vi "Repair.vi"() -> ()   [LabVIEW 2019]
uses:
  Control 3.ctl
  Control 1.ctl
  <vilib>/Analysis/3filter.llb/Filter Passband Type.ctl
  <vilib>/Analysis/5stat.llb/RMS (DBL).vi
  <vilib>/Waveform/WDTOps.llb/WDT Append Waveforms DBL.vi
  <vilib>/Analysis/3filter.llb/Butterworth Filter (DBL).vi
  <vilib>/Analysis/NI_AALPro.lvlib
  <vilib>/Analysis/NI_AALBase.lvlib
panel:
  out "1/x":dbl
  out "Numeric":dbl
  out "XY Graph":cluster{dbl[], "Vstupní pole":dbl[]}(graph)
  out "Prubehy RMS":cluster{"rms value":dbl}(graph)
  out "Perioda ze spektra.":dbl
  out "Urms":dbl format="%0.2f"
  out "Perioda z pruchodu nulou.":dbl
  out "Frekvence z pruchodu nulou.":dbl
  out "Frekvence ze spektra.":i32
  out "Spektrum prevzorkovaneho signalu":cluster{dbl[], dbl[]}(graph)
  out "Prevzorkovany signal":waveform(dbl)(graph)
  in  "Napetovy treshold":dbl=10.0
  in  "Sirka okna (ms)":i32(listbox)=1
  in  "Offset":dbl format="%0.2p"
  in  "Amplituda sumu":T1
  in  "Amplituda":dbl=1.0 format="%0.2p"
  in  "Frekvence":dbl=10.0 format="%0.2p"
  out "Signal z generatoru":waveform(dbl)(graph)
  in  "stop":bool
  # "Parametry generatoru signalu"
  # "Hide!"
  # "Parametry navzorkovaneho signalu"
  # "Parametry prevzorkovaneho signalu"
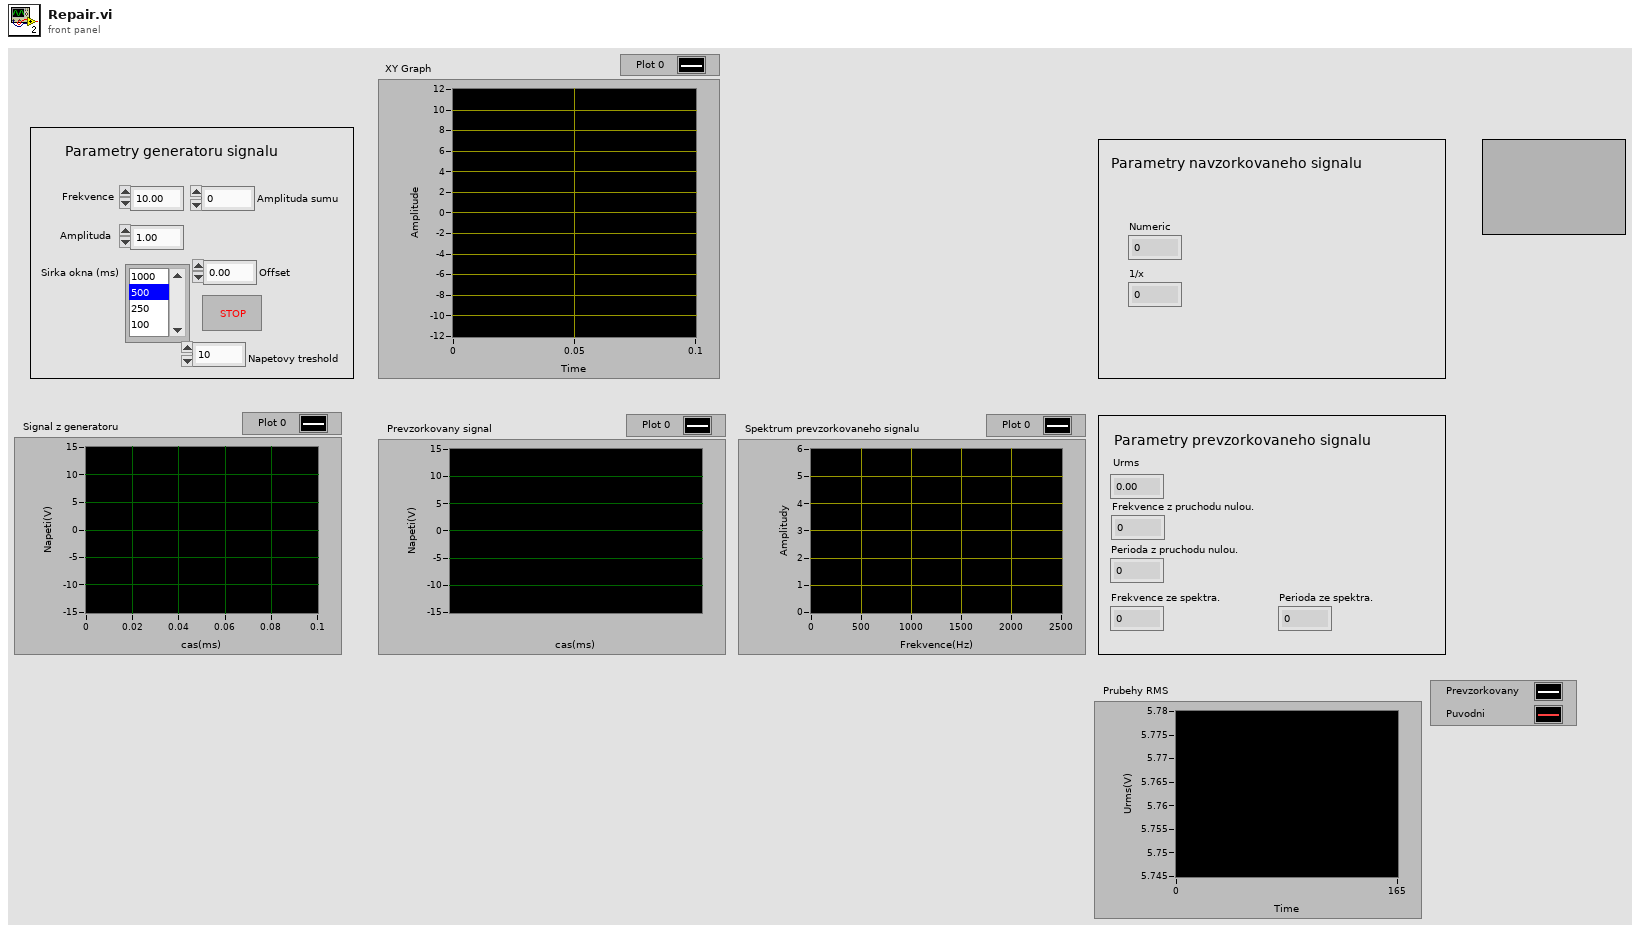
[diagram p1: front panel]
types:
  T1 = typedef "Control 3.ctl" = dbl
  T2 = enum16{"open", "open or create", "create or replace", "create", "open (read-only)"}
  T3 = cluster{"Waveform":waveform(dbl), "Waveform":waveform(dbl), "Waveform":waveform(dbl), "seconds since 1Jan1904":timestamp, bool, bool}
  T4 = typedef "Control 1.ctl" = dbl
  T5 = cluster{"name (unnamed)":string, "Variant":variant}
  T6 = typedef "NI_AALBase.lvlib/Filter Passband Type.ctl" = enum32{"Lowpass", "Highpass", "Bandpass", "Bandstop"}
  T7 = cluster{waveform(dbl), waveform(dbl), waveform(dbl), "seconds since 1Jan1904":timestamp, bool, bool}
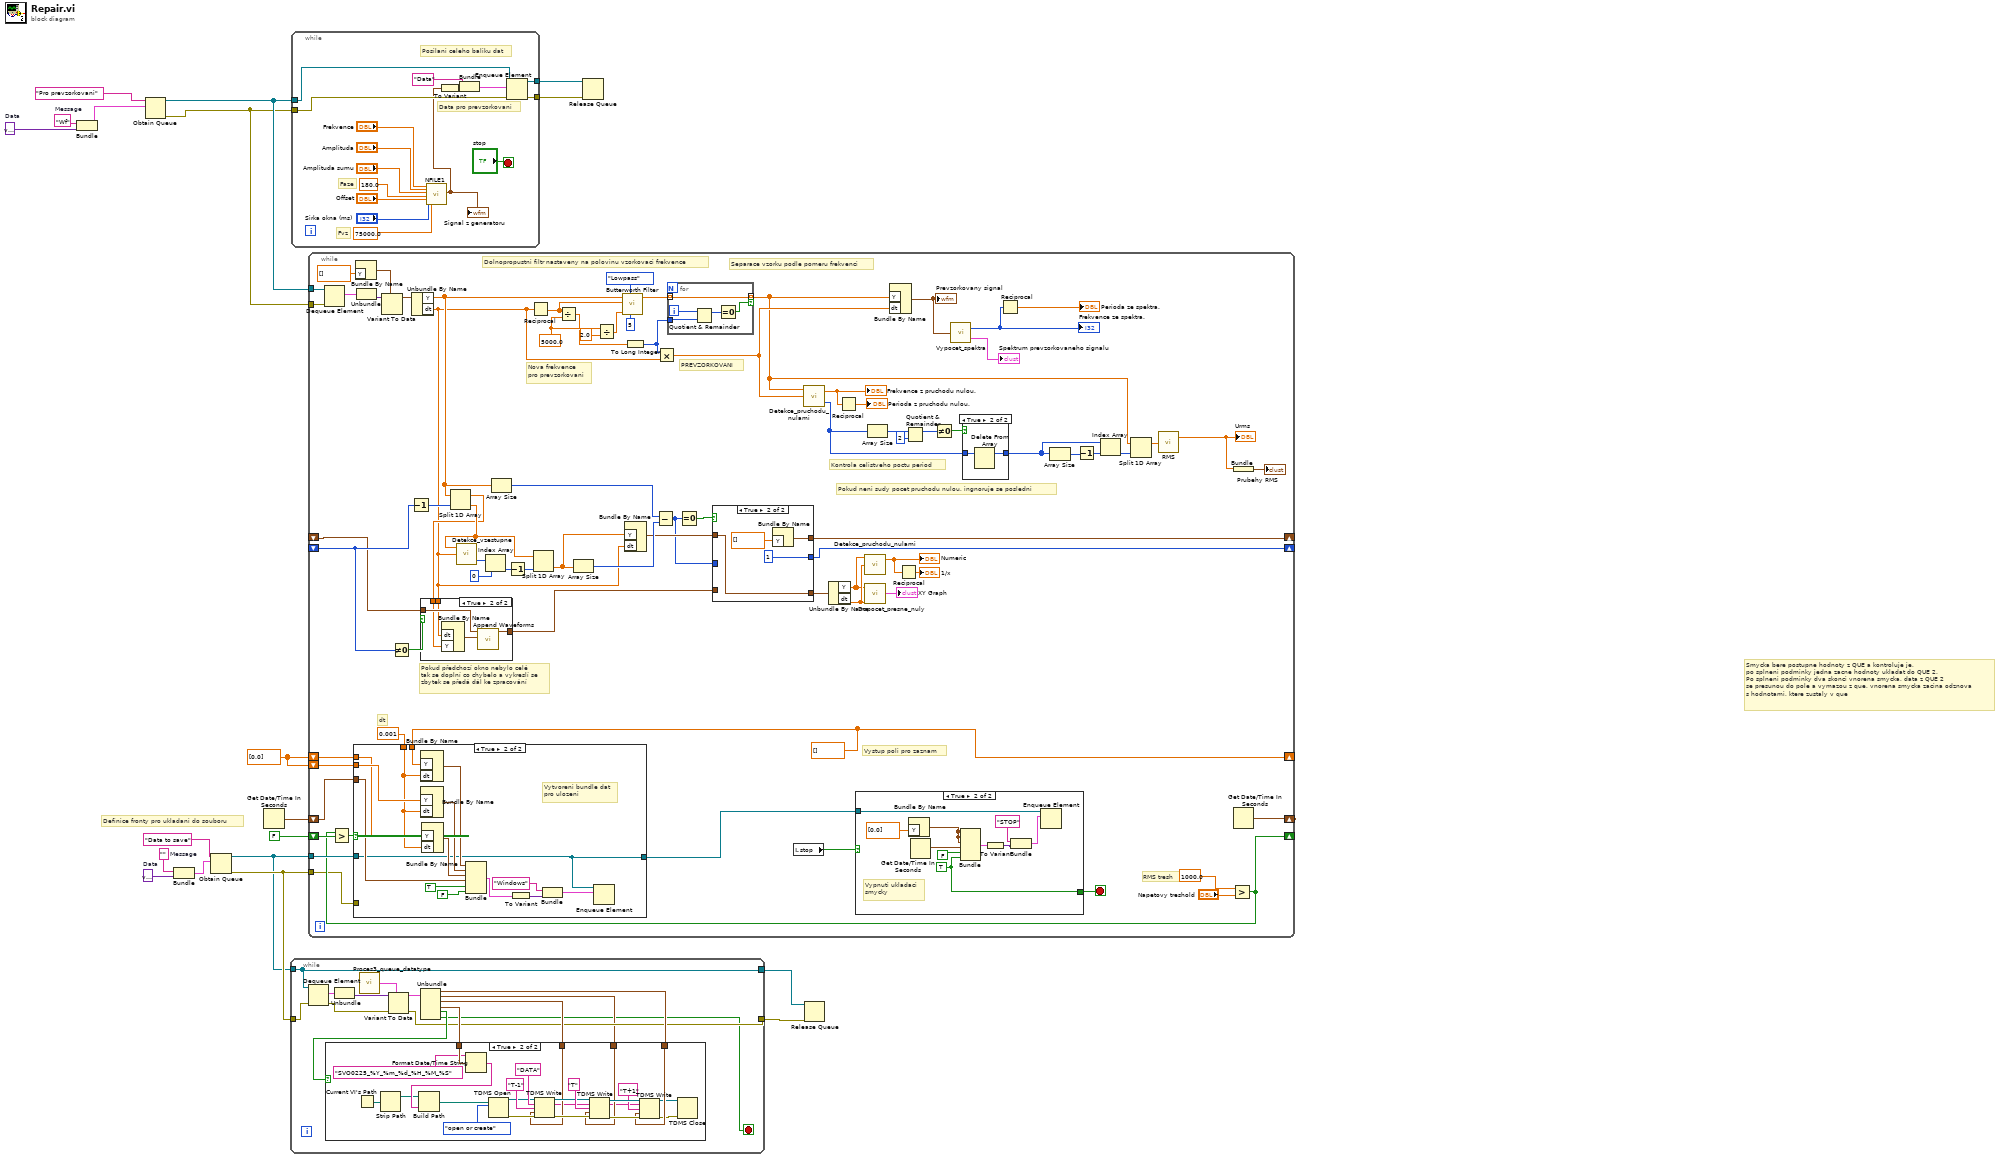
[diagram p0: block diagram]
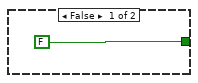
[diagram p5: hidden frame]
diagram:
  w4 = dbl[] [0.0]
  w3 = variant  # Data
  w8 = "Wf"  # Message
  w17 = variant  # Data
  w18 = ""  # Message
  # "Definice fronty pro ukladani do souboru"
  # "Smycka bere postupne hodnoty z QUE a kontroluje je,\npo splneni podminky jedna zacne hodnoty ukladat do QUE 2.\nPo splneni podminky dva skonci vnorena smycka, data z QUE 2 \nse presunou do pole a vymazou z que, vnorena smycka zacina odznova\ns hodnotami, ktere zustaly v que"
  n1 = Bundle("Message"=w8, "Data"=w3) -> (w7:cluster{"Message":string, "Data":variant})  [unwired: 1 in]
  n2 = Obtain Queue(name (unnamed)="Pro prevzorkovani", element data type=w7) -> (queue out=w10:refnum<queue>, error out=w9:errorcluster)  [unwired: 3 in, 1 out]
  n3 = Bundle("Message"=w18, "Data"=w17) -> (w16:cluster{"Message":string, "Data":variant})  [unwired: 1 in]
  n4 = Obtain Queue(name (unnamed)="Data to save", element data type=w16) -> (queue out=w13:refnum<queue>, error out=w14:errorcluster)  [unwired: 3 in, 1 out]
  n5 = Get Date/Time In Seconds() -> (seconds since 1Jan1904=w5:timestamp)
  n6 = while {
    tunnel: w14 -> [w24]
    tunnel: w13 -> [w29]
    tunnel: [w29] -> w12
    tunnel: [w22] -> w11
    stop <- w20 stop-if-true
    n7 = Dequeue Element(queue=w29, error in (no error)=w24) -> (element=w33:cluster{"Message":string, "Data":variant}, error out=w23:errorcluster)  [unwired: 1 in, 2 out]
    n8 = Unbundle(w33) -> ("Data"=w32:variant)  [unwired: 1 out]
    n9 = call "Proces3_queue_datatype.vi"() -> ("output cluster"=w31:T3)  [unwired: 1 in]
    n10 = Variant To Data(error in=w23, type=w31, Variant=w32) -> (data=w30:T3, error out=w22:errorcluster)
    n11 = Unbundle(w30) -> ("Waveform"=w28:waveform(dbl), "Waveform"=w21:waveform(dbl), "Waveform"=w25:waveform(dbl), "seconds since 1Jan1904"=w27:timestamp, w26:bool, w20:bool)
    n12 = case shown="True" w26 {
      tunnel: w28 -> [_ w46]
      tunnel: w27 -> [_ w45]
      tunnel: w25 -> [_ w39]
      tunnel: w21 -> [_ w38]
      frame False {
      }
      frame True {
        n13 = Current VI's Path() -> (path=w57:path)
        n14 = Strip Path(path=w57) -> (stripped path=w34:path)  [unwired: 1 out]
        n15 = Format Date/Time String(time format string (%c)="SVO0225_%Y_%m_%d_%H_%M_%S", seconds (now)=w45) -> (date/time string=w56:string)  [unwired: 1 in]
        n16 = Build Path(base path=w34, name or relative path=w56) -> (appended path=w55:path)
        n17 = TDMS Open(10:T2."open or create" ("operation (0:open)"), 11:w55) -> (0:w50:errorcluster, 3:w51:refnum<k34>)  [unwired: 5 in]
        n18 = TDMS Write(0:w51, 5:"DATA" ("group name in (Untitled)"), 7:"T-1", 9:w39, 11:w50) -> (4:w40:refnum<k34>, 6:w37:string, 15:w49:errorcluster)  [unwired: 1 in, 1 out]
        n19 = TDMS Write(0:w40, 5:w37, 7:"T", 9:w38, 11:w49) -> (4:w41:refnum<k34>, 6:w35:string, 15:w47:errorcluster)  [unwired: 1 in, 1 out]
        n20 = TDMS Write(0:w41, 5:w35, 7:"T+1", 9:w46, 11:w47) -> (4:w43:refnum<k34>, 15:w44:errorcluster)  [unwired: 1 in, 2 out]
        n21 = TDMS Close(8:w44, 11:w43) -> ()  [unwired: 2 out]
      }
    }
  }
  n22 = while {
    tunnel: w10 -> [w65]
    tunnel: w9 -> [w64]
    tunnel: [w59] -> w2
    tunnel: [w58] -> w1
    stop <- "stop" stop-if-true
    # "Posilani celeho baliku dat"
    # "Data pro prevzorkovani"
    # "Fvz"
    # "Faze"
    n23 = call "NFILE1.vi"("Frekvence"="Frekvence", "Amplituda"="Amplituda", "Amplituda sumu"="Amplituda sumu", "Fáze"=180.0, "Offset"="Offset", "Sirka okna (ms)"="Sirka okna (ms)", "Fvz"=T4 75000.0) -> ("Waveform Graph"=w61:waveform(dbl))  [unwired: 12 in]
    "Signal z generatoru" <- w61
    n24 = To Variant(anything=w61) -> (Variant=w62:variant)
    n25 = Bundle("name (unnamed)"="Data", "Variant"=w62) -> (w63:T5)  [unwired: 1 in]
    n26 = Enqueue Element(queue=w65, element=w63, error in (no error)=w64) -> (queue out=w59:refnum<queue>, error out=w58:errorcluster)  [unwired: 1 in, 1 out]
  }
  n27 = while {
    shift-right: [w104] -> _
    shift-left: w4 -> [w150]
    shift-left: w4 -> [w149]
    shift-right: [w114] -> _
    shift-left: FALSE -> [w147]
    tunnel: w13 -> [w151]
    tunnel: w14 -> [w108]
    tunnel: w10 -> [w146]
    tunnel: w9 -> [w145]
    shift-right: [w110] -> _
    shift-left: w5 -> [w109]
    shift-right: [w90] -> _
    shift-left: _ -> [w86]
    shift-right: [w89] -> _
    shift-left: _ -> [w84]
    stop <- w107 stop-if-true
    w104 = dbl[] []
    w136 = T4 5000.0 ("Fvz")
    # "Pokud předchozí okno nebylo celé\ntak se doplní co chybelo a vykreslí se\nzbytek se předá dál ke zpracování"
    # "dt"
    # "RMS tresh"
    # "Vystup poli pro zaznam"
    # "PREVZORKOVANI"
    # "Pokud neni sudy pocet pruchodu nulou, ingnoruje se posledni"
    # "Kontrola celistveho poctu period"
    # "Separace vzorku podle pomeru frekvenci"
    # "Dolnopropustni filtr nastaveny na polovinu vzorkovaci frekvence"
    # "Nova frekvence\npro prevzorkovani"
    n28 = Dequeue Element(queue=w146, error in (no error)=w145) -> (element=w144:cluster{"Message":string, "Data":variant})  [unwired: 1 in, 3 out]
    n29 = Bundle By Name("Y"=dbl[] []) -> (w142:waveform(dbl))  [unwired: 1 in]
    n30 = Unbundle(w144) -> ("Data"=w143:variant)  [unwired: 1 out]
    n31 = Variant To Data(type=w142, Variant=w143) -> (data=w141:waveform(dbl))  [unwired: 1 in, 1 out]
    n32 = Not Equal To 0?(x=w86) -> (x != 0?=w80:bool)
    n33 = Decrement(x=w86) -> (x-1=w85:i32)
    n34 = Unbundle By Name(w141) -> ("Y"=w88:dbl[], "dt"=w82:dbl)
    n35 = Split 1D Array(array=w88, index=w85) -> (first subarray=w83:dbl[], second subarray=w87:dbl[])
    n36 = case shown="True" w80 {
      tunnel: w84 -> [w153 w158]
      tunnel: w83 -> [_ w157]
      tunnel: w82 -> [_ w156]
      tunnel: [w153 w154] -> w81
      frame False {
      }
      frame True {
        n37 = Bundle By Name("dt"=w156, "Y"=w157) -> (w155:waveform(dbl))  [unwired: 1 in]
        n38 = call-poly <vilib>:"Append Waveforms.vi"("waveform B"=w155, "waveform A"=w158) -> ("waveform out"=w154:waveform(dbl))  [unwired: 8 in, 1 out]
      }
    }
    n39 = call "Detekce_vzestupne.vi"("dt 2"=w82, "array"=w87) -> ("Pole indexu pruchodu nulou"=w99:i32[])  [unwired: 1 in, 1 out]
    n40 = Index Array(array=w99, index=0) -> (element=w98:i32)
    n41 = Array Size(array=w88) -> (size(s)=w95:i32)
    n42 = Decrement(x=w98) -> (x-1=w97:i32)
    n43 = Reciprocal(x=w82) -> (1/x=w135:dbl)
    n44 = Split 1D Array(array=w87, index=w97) -> (second subarray=w96:dbl[])  [unwired: 1 out]
    n45 = Divide(x=w135, y=w136) -> (x/y=w133:T4)
    n46 = Array Size(array=w96) -> (size(s)=w94:i32)
    n47 = Divide(x=w136, y=2.0) -> (x/y=w139:T4)
    n48 = call-poly <vilib>:"Butterworth Filter.vi"("order"=5, "filter type"=Filter_Passband_Type."Lowpass", "low cutoff freq: fl"=w139, "sampling freq: fs"=w135, "X"=w88) -> ("Filtered X"=w134:dbl[])  [unwired: 3 in, 1 out]
    n49 = Bundle By Name("Y"=w96, "dt"=w82) -> (w92:waveform(dbl))  [unwired: 1 in]
    n50 = To Long Integer(number=w133) -> (32bit integer=w132:i32)
    n51 = Subtract(x=w95, y=w94) -> (x-y=w91:i32)
    n52 = Multiply(x=w132, y=w82) -> (x*y=w128:dbl)
    n53 = for {
      tunnel: w134 -> [w197] mode=indexing
      tunnel: w132 -> [w199]
      tunnel: [w197] -> w116 mode=indexing if=w196
      i -> [w200]
      n54 = Quotient & Remainder(x=w200, y=w199) -> (x-y*floor(x/y)=w198:i32)  [unwired: 1 out]
      n55 = Equal To 0?(x=w198) -> (x = 0?=w196:bool)
    }
    n56 = Equal To 0?(x=w91) -> (x = 0?=w93:bool)
    n57 = case shown="True" w93 {
      tunnel: w92 -> [w160 w164]
      tunnel: w91 -> [w161 _]
      tunnel: [w161 1] -> w90
      tunnel: [w160 w162] -> w89
      tunnel: [w159 w164] -> w79
      tunnel: w81 -> [w159 _]
      frame False {
      }
      frame True {
        n58 = Bundle By Name("Y"=dbl[] []) -> (w162:waveform(dbl))  [unwired: 1 in]
      }
    }
    n59 = local read "stop"() -> (w106:bool)
    n60 = call "Detekce_pruchodu_nulami.vi"("dt 2"=w128, "array"=w116) -> ("Pole indexu pruchodu nulou"=w121:i32[], "Numeric"=w126:dbl)  [unwired: 1 in]
    "Frekvence z pruchodu nulou." <- w126
    n61 = Unbundle By Name(w79) -> ("Y"=w76:dbl[], "dt"=w77:dbl)
    n62 = Reciprocal(x=w126) -> (1/x=→"Perioda z pruchodu nulou.":dbl)
    n63 = call "Detekce_pruchodu_nulami.vi"("dt 2"=w77, "array"=w76) -> ("Numeric"=w75:dbl)  [unwired: 1 in, 1 out]
    "Numeric" <- w75
    n64 = call "Dopocet_presne_nuly.vi"("dt"=w77, "Vstupní pole"=w76) -> ("XY Graph"=→"XY Graph":cluster{dbl[], "Vstupní pole":dbl[]})  [unwired: 9 in]
    n65 = Array Size(array=w121) -> (size(s)=w124:i32)
    n66 = Bundle By Name("Y"=w116, "dt"=w128) -> (w130:waveform(dbl))  [unwired: 1 in]
    "Prevzorkovany signal" <- w130
    n67 = Reciprocal(x=w75) -> (1/x=→"1/x":dbl)
    n68 = Quotient & Remainder(x=w124, y=2) -> (x-y*floor(x/y)=w125:i32)  [unwired: 1 out]
    n69 = Not Equal To 0?(x=w125) -> (x != 0?=w122:bool)
    n70 = call "Vypocet_spektra.vi"("waveform"=w130) -> ("Frekvence"=w112:i32, "XY Graph"=→"Spektrum prevzorkovaneho signalu":cluster{dbl[], dbl[]})
    "Frekvence ze spektra." <- w112
    n71 = case shown="True" w122 {
      tunnel: w121 -> [w193 w195]
      tunnel: [w193 w194] -> w118
      frame False {
      }
      frame True {
        n72 = Delete From Array(array=w195) -> (array with subset deleted=w194:i32[])  [unwired: 2 in, 1 out]
      }
    }
    n73 = Reciprocal(x=w112) -> (1/x=→"Perioda ze spektra.":dbl)
    n74 = Array Size(array=w118) -> (size(s)=w120:i32)
    n75 = Decrement(x=w120) -> (x-1=w119:i32)
    n76 = Index Array(array=w118, index=w119) -> (element=w117:i32)
    n77 = Split 1D Array(array=w116, index=w117) -> (first subarray=w115:dbl[])  [unwired: 1 out]
    n78 = call-poly <vilib>:"RMS.vi"("X"=w115) -> ("rms value"=w111:dbl)  [unwired: 1 out]
    "Urms" <- w111
    n79 = Greater?(x=1000.0, y="Napetovy treshold") -> (0:w114:bool)
    n80 = Greater?(x=w114, y=w147) -> (0:w148:bool)
    n81 = case shown="True" w148 {
      tunnel: w151 -> [w177 w179]
      tunnel: w150 -> [_ w185]
      tunnel: w149 -> [_ w186]
      tunnel: w104 -> [_ w187]
      tunnel: w109 -> [_ w188]
      tunnel: w108 -> [_ _]
      tunnel: [w177 w179] -> w105
      tunnel: 0.001 -> [_ w178]
      frame False {
      }
      frame True {
        # "Vytvoreni bundle dat\npro ulozeni"
        n82 = Bundle By Name("Y"=w187, "dt"=w178) -> (w182:waveform(dbl))  [unwired: 1 in]
        n83 = Bundle By Name("Y"=w186, "dt"=w178) -> (w183:waveform(dbl))  [unwired: 1 in]
        n84 = Bundle By Name("Y"=w185, "dt"=w178) -> (w184:waveform(dbl))  [unwired: 1 in]
        n85 = Bundle(w182, w183, w184, "seconds since 1Jan1904"=w188, TRUE, FALSE) -> (w190:T7)  [unwired: 1 in]
        n86 = To Variant(anything=w190) -> (Variant=w191:variant)
        n87 = Bundle("Windows", "Variant"=w191) -> (w189:cluster{string, "Variant":variant})  [unwired: 1 in]
        n88 = Enqueue Element(queue=w179, element=w189) -> ()  [unwired: 2 in, 3 out]
      }
    }
    n89 = case shown="True" w106 {
      tunnel: [FALSE w173] -> w107
      tunnel: w105 -> [_ w171]
      frame False {
      }
      frame True {
        w173 = TRUE
        # "Vypnuti ukladaci\nsmycky"
        n90 = Bundle By Name("Y"=dbl[] [0.0]) -> (w176:waveform(dbl))  [unwired: 1 in]
        n91 = Get Date/Time In Seconds() -> (seconds since 1Jan1904=w175:timestamp)
        n92 = Bundle(w176, w176, w176, "seconds since 1Jan1904"=w175, FALSE, w173) -> (w169:T7)  [unwired: 1 in]
        n93 = To Variant(anything=w169) -> (Variant=w170:variant)
        n94 = Bundle("STOP", "Variant"=w170) -> (w167:cluster{string, "Variant":variant})  [unwired: 1 in]
        n95 = Enqueue Element(queue=w171, element=w167) -> ()  [unwired: 2 in, 3 out]
      }
    }
    n96 = Bundle("rms value"=w111) -> (→"Prubehy RMS":cluster{"rms value":dbl})  [unwired: 1 in]
    n97 = Get Date/Time In Seconds() -> (seconds since 1Jan1904=w110:timestamp)
  }
  n98 = Release Queue(queue=w2, error in (no error)=w1) -> ()  [unwired: 1 in, 3 out]
  n99 = Release Queue(queue=w12, error in (no error)=w11) -> ()  [unwired: 1 in, 3 out]
